vi "IPS Read Target Current.vi"(4 "Error In":errorcluster={"status"=FALSE, "code"=1073676294, "source"="VISA Read in Prologix USB GPIB Command.vi"}, 7 "VISA resource name":refnum<visa-resource-name>="COM3") -> (0 "Error Out":errorcluster={"status"=FALSE, "code"=1073676294, "source"="VISA Read in Prologix_GPIB_Sample.vi"}, 2 "Set Point (A)":dbl, 3 "VISA resource name 2":refnum<visa-resource-name>="COM3")   [LabVIEW 2016, in "IPS-120.lvlib"]
uses:
  IPS-120.lvlib
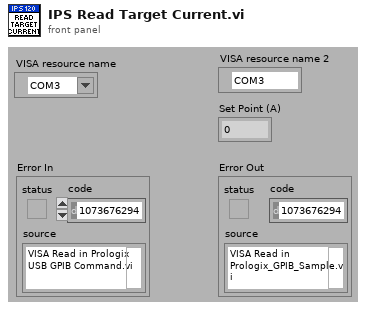
[diagram p1: front panel]
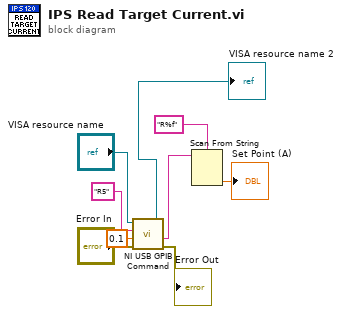
[diagram p0: block diagram]
diagram:
  n1 = call "NI USB GPIB Command.vi"("Error In"="Error In", "Wait for instrument to respond (s)"=0.1, "String to Send"="R5", "VISA resource name"="VISA resource name") -> ("Error Out"=→"Error Out":errorcluster, "Return String from Device (Not all commands return a String)"=w4:string, "VISA resource name"=→"VISA resource name 2":refnum<visa-resource-name>)  [unwired: 1 out]
  n2 = Scan From String(format string="R%f", input string=w4) -> (output 1=→"Set Point (A)":dbl)  [unwired: 2 in, 4 out]
